vi "PAN_MacroCmd.vi"(6 "timeout in ms (-1)":i32=-1, 8 "error in (no error)":errorcluster, 11 "Command":string) -> (0 "error out":errorcluster, 3 "response":string)   [LabVIEW 2016]
panel:
  in  "Cluster":T1
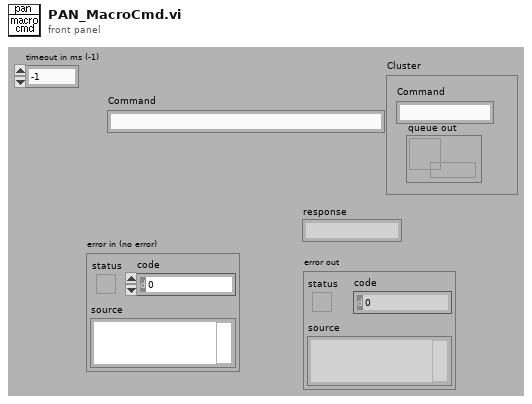
[diagram p1: front panel]
types:
  T1 = cluster{"Command ":string, "queue out":refnum<queue>}
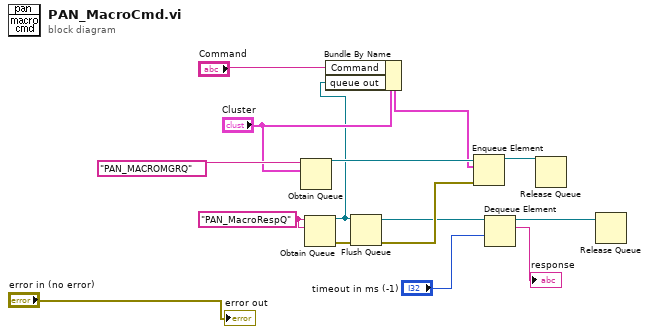
[diagram p0: block diagram]
diagram:
  w4 = "PAN_MacroRespQ" ("name (unnamed)")
  n1 = Obtain Queue(name (unnamed)="PAN_MACROMGRQ", element data type="Cluster") -> (queue out=w15:refnum<queue>)  [unwired: 3 in, 2 out]
  n2 = Obtain Queue(name (unnamed)=w4, element data type=w4) -> (queue out=w3:refnum<queue>, error out=w8:errorcluster)  [unwired: 3 in, 1 out]
  n3 = Bundle By Name(cluster="Cluster", "Command"="Command", "queue out"=w3) -> (w10:T1)
  n4 = Flush Queue(queue=w3, error in (no error)=w8) -> (queue out=w6:refnum<queue>, error out=w7:errorcluster)  [unwired: 1 out]
  n5 = Enqueue Element(queue=w15, element=w10, error in (no error)=w7) -> (queue out=w14:refnum<queue>)  [unwired: 3 out]
  n6 = Dequeue Element(queue=w6, timeout in ms (-1)="timeout in ms (-1)") -> (queue out=w5:refnum<queue>, element=→"response":string)  [unwired: 1 in, 2 out]
  n7 = Release Queue(queue=w14) -> ()  [unwired: 1 in, 4 out]
  n8 = Release Queue(queue=w5) -> ()  [unwired: 1 in, 4 out]
  "error out" <- "error in (no error)"
